vi "全局变量.vi"() -> ()   [LabVIEW 2011]
panel:
  in  "同步码？":bool
  in  "原始数据":i32
  in  "按下次数":i32
  in  "完成？":bool
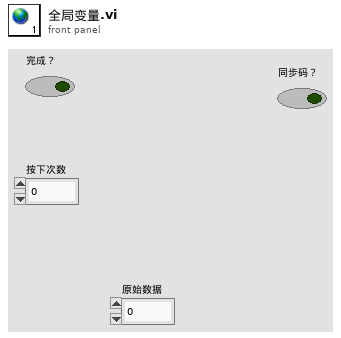
[diagram p1: front panel]
diagram:
